vi "EvaluateOperatingStates.vi"(7 "data group":string, 8 "error in (no error)":errorcluster, 9 "map":T1, 10 "config in":T2, 11 "Qbus in":refnum<class "Qbus.lvclass">) -> (0 "error out":errorcluster, 2 "config out":T2, 3 "Qbus out":refnum<class "Qbus.lvclass">)   [LabVIEW 2017, in "OpState.lvlib"]
uses:
  <vilib>/addons/InsightCM/Devices/Shared/Common/OpState/OpState.lvlib
  <vilib>/addons/InsightCM/Devices/Shared/Common/OpState/controls/config.ctl
  <vilib>/addons/Qbus/Qbus.lvclass
  <vilib>/addons/PointValueMap/controls/PointMap.ctl
  <vilib>/addons/InsightCM/Devices/Shared/Common/OpState/controls/ConditionType.ctl
  <vilib>/addons/PointValueMap/subVIs/Point_Write_string.vi
  <vilib>/addons/PointValueMap/PointValueMap.lvlib
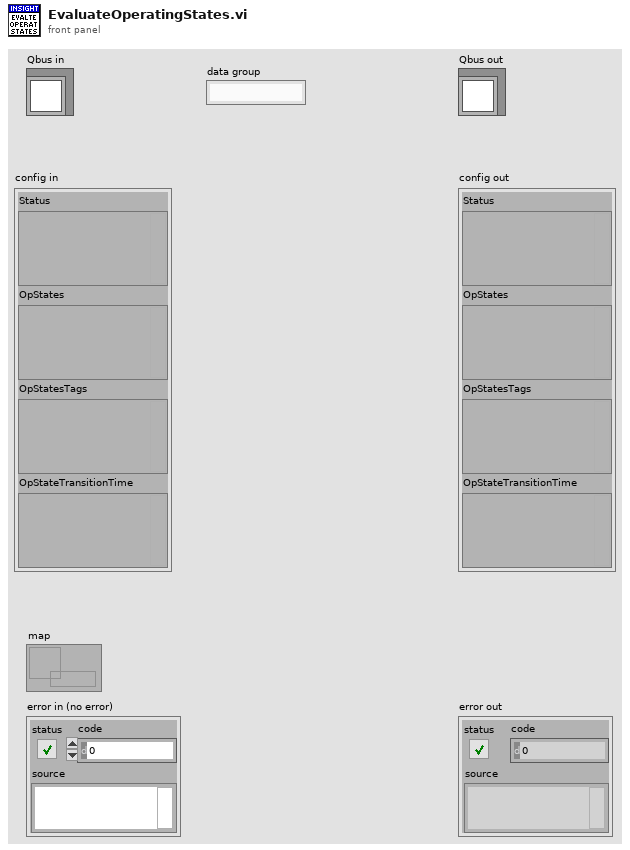
[diagram p1: front panel]
types:
  T1 = typedef "PointValueMap.lvlib/PointMap.ctl" = refnum<data-value>
  T2 = typedef "OpState.lvlib/config.ctl" = cluster{"Status":variant, "OpStates":variant, "OpStatesTags":variant, "OpStateTransitionTime":variant}
  T3 = typedef "OpState.lvlib/ConditionType.ctl" = enum16{"Enter", "Exit"}
  T4 = typedef "Trigger.lvlib/TriggerCondition.ctl" = cluster{"Condition":T5, "LatchValue":string, "LatchTime":timestamp}
  T5 = typedef "Condition.ctl" = cluster{"Source":string, "Type":string, "Operator":string, "CompareTo":string, "DwellSeconds":dbl}
  T6 = typedef "OpState.lvlib/TriggerOperatingState.ctl" = cluster{"Id":string, "Name":string, "Properties":T7[], "EnterExpression":string, "EnterConditions":T4[], "ExitExpression":string, "ExitConditions":T4[]}
  T7 = typedef "KeyValuePair.ctl" = cluster{"Key":string, "Value":string}
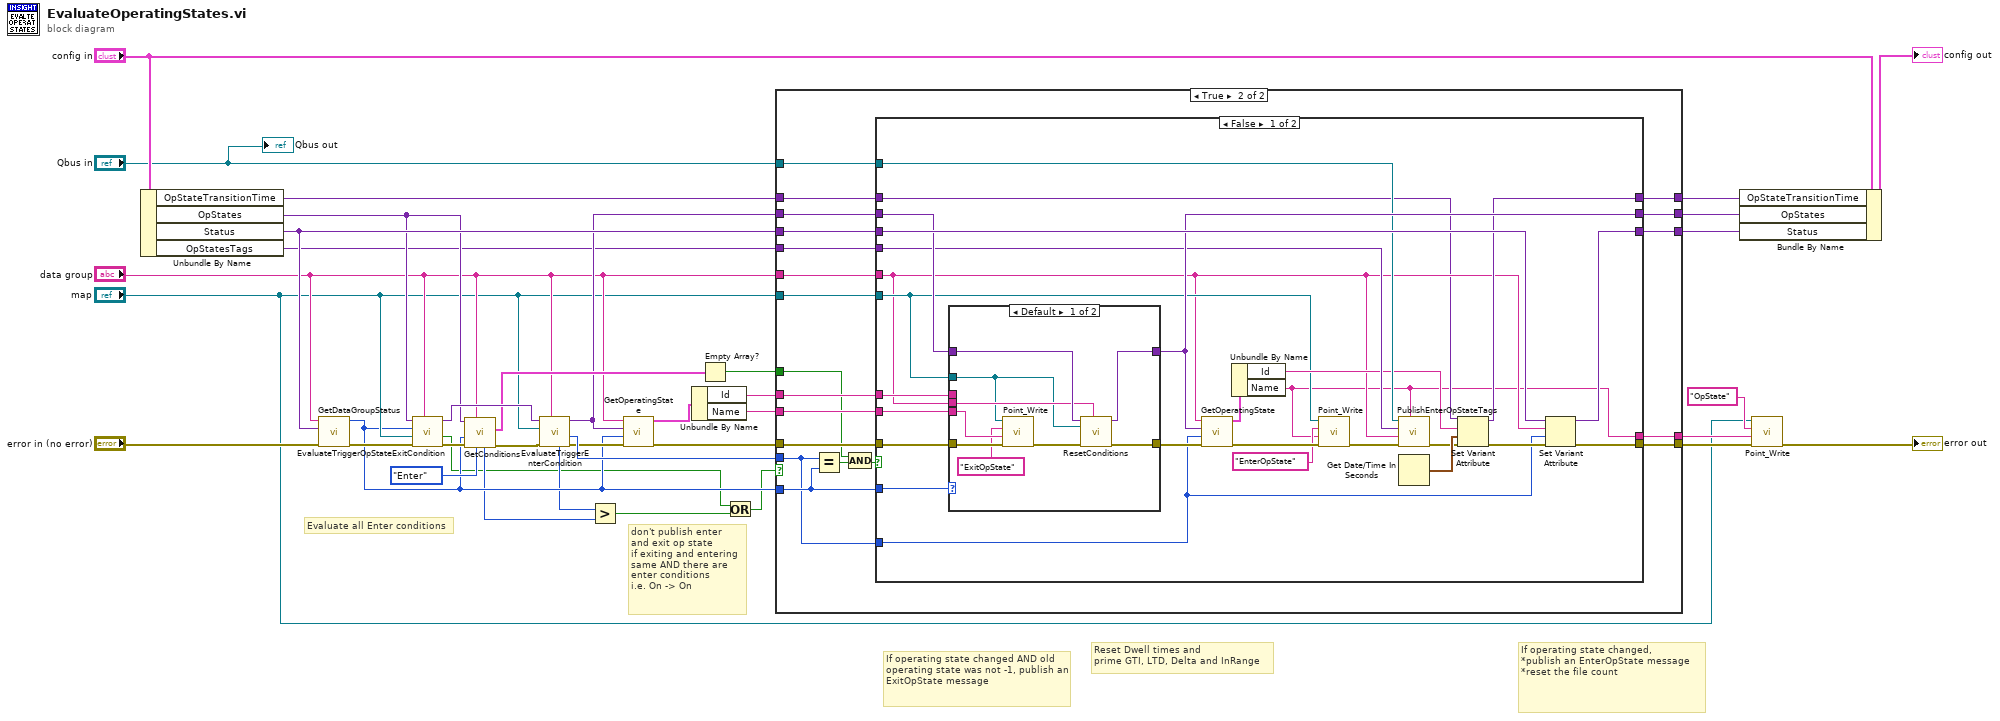
[diagram p0: block diagram]
diagram:
  # "don't publish enter\nand exit op state\nif exiting and entering\nsame AND there are\nenter conditions\ni.e. On -> On"
  # "Reset Dwell times and \nprime GTI, LTD, Delta and InRange"
  # "Evaluate all Enter conditions"
  # "If operating state changed, \n*publish an EnterOpState message\n*reset the file count"
  # "If operating state changed AND old operating state was not -1, publish an ExitOpState message"
  n1 = Unbundle By Name("config in") -> ("OpStateTransitionTime"=w19:variant, "OpStates"=w17:variant, "Status"=w30:variant, "OpStatesTags"=w8:variant)
  n2 = call <vilib>:"GetDataGroupStatus.vi"("error in"="error in (no error)", "status"=w30, "data group"="data group") -> ("error out"=w28:errorcluster, "CurrentOpState"=w7:i32)  [unwired: 7 in]
  n3 = call <vilib>:"EvaluateTriggerOpStateExitCondition.vi"("data group"="data group", "error in"=w28, "map"="map", "current op state"=w7, "operating states in"=w17) -> ("error out"=w13:errorcluster, "exit"=w3:bool, "operating states out"=w33:variant)  [unwired: 4 in]
  n4 = call <vilib>:"GetConditions.vi"("condition type"=ConditionType."Enter", "data group"="data group", "error in (no error)"=w13, "operating state"=w7, "operating states in"=w17) -> ("error out"=w12:errorcluster, "conditions"=w15:T4[], "weight"=w5:i32)  [unwired: 2 in, 2 out]
  n5 = call <vilib>:"EvaluateTriggerEnterCondition.vi"("data group"="data group", "error in"=w12, "map"="map", "operating states in"=w33) -> ("error out"=w23:errorcluster, "new operating state"=w32:i32, "operating states out"=w11:variant, "weight"=w6:i32)  [unwired: 4 in]
  n6 = Greater?(x=w6, y=w5) -> (0:w4:bool)
  n7 = call <vilib>:"GetOperatingState.vi"("error in"=w23, "index"=w7, "operating states"=w11, "data group"="data group") -> ("error out"=w1:errorcluster, "operating state"=w22:T6)  [unwired: 6 in]
  n8 = Unbundle By Name(w22) -> ("Id"=w20:string, "Name"=w21:string)
  n9 = Empty Array?(array=w15) -> (empty?=w14:bool)
  n10 = Or(x=w3, y=w4) -> (x .or. y?=w2:bool)
  n11 = case shown="True" w2 {
    tunnel: w1 -> [w40 w55]
    tunnel: [w40 w62] -> w26
    tunnel: "Qbus in" -> [_ w59]
    tunnel: w11 -> [w41 w54]
    tunnel: "data group" -> [_ w61]
    tunnel: w7 -> [_ w60]
    tunnel: w30 -> [w42 w58]
    tunnel: [w42 w57] -> w34
    tunnel: [w41 w56] -> w35
    tunnel: w32 -> [_ w53]
    tunnel: "map" -> [_ w52]
    tunnel: [w39 w50] -> w24
    tunnel: w21 -> [w39 w51]
    tunnel: w8 -> [_ w49]
    tunnel: w20 -> [_ w48]
    tunnel: w19 -> [w38 w47]
    tunnel: [w38 w46] -> w18
    tunnel: w14 -> [_ w43]
    frame False {
    }
    frame True {
      n12 = Equal?(x=w53, y=w60) -> (x = y?=w44:bool)
      n13 = Compound Arithmetic op=AND(w43, w44) -> (w45:bool)
      n14 = case shown="False" w45 {
        tunnel: w55 -> [w88 w103]
        tunnel: [w82 w103] -> w62
        tunnel: w61 -> [w65 _]
        tunnel: w54 -> [w81 w104]
        tunnel: w60 -> [w87 _]
        tunnel: w59 -> [w74 _]
        tunnel: w53 -> [w66 _]
        tunnel: w58 -> [w84 w102]
        tunnel: [w83 w102] -> w57
        tunnel: [w80 w104] -> w56
        tunnel: w52 -> [w68 _]
        tunnel: w51 -> [w79 w101]
        tunnel: [w63 w101] -> w50
        tunnel: w49 -> [w75 _]
        tunnel: w48 -> [w76 _]
        tunnel: w47 -> [w64 w100]
        tunnel: [w69 w100] -> w46
        frame False {
          n15 = case shown="Default" w87 {
            tunnel: w88 -> [w93 w99]
            tunnel: w65 -> [w94 _]
            tunnel: w81 -> [w96 w98]
            tunnel: [w97 w99] -> w86
            tunnel: [w95 w98] -> w80
            tunnel: w68 -> [w90 _]
            tunnel: w79 -> [w92 _]
            tunnel: w76 -> [_ _]
            frame Default {
              n16 = call-poly <vilib>:"Point_Write.vi"("Error In"=w93, "Value"=w92, "Tag"="ExitOpState", "Map"=w90) -> ("Error Out"=w89:errorcluster)  [unwired: 6 in, 1 out]
              n17 = call <vilib>:"ResetConditions.vi"("data group"=w94, "error in (no error)"=w89, "map"=w90, "operating states in"=w96) -> ("error out"=w97:errorcluster, "operating states out"=w95:variant)  [unwired: 6 in]
            }
            frame -1 {
            }
          }
          n18 = call <vilib>:"GetOperatingState.vi"("error in"=w86, "index"=w66, "operating states"=w80, "data group"=w65) -> ("error out"=w78:errorcluster, "operating state"=w85:T6)  [unwired: 6 in]
          n19 = Unbundle By Name(w85) -> ("Id"=w73:string, "Name"=w63:string)
          n20 = call-poly <vilib>:"Point_Write.vi"("Error In"=w78, "Value"=w63, "Tag"="EnterOpState", "Map"=w68) -> ("Error Out"=w67:errorcluster)  [unwired: 6 in, 1 out]
          n21 = call <vilib>:"PublishEnterOpStateTags.vi"("op state"=w63, "error in (no error)"=w67, "data group name"=w65, "operating states tags"=w75, "Qbus in"=w74) -> ("error out"=w71:errorcluster)  [unwired: 6 in]
          n22 = Get Date/Time In Seconds() -> (seconds since 1Jan1904=w72:timestamp)
          n23 = Set Variant Attribute(Variant=w64, name=w73, value=w72, error in=w71) -> (Variant out=w69:variant, error out=w70:errorcluster)  [unwired: 1 out]
          n24 = Set Variant Attribute(Variant=w84, name=w65, value=w66, error in=w70) -> (Variant out=w83:variant, error out=w82:errorcluster)  [unwired: 1 out]
        }
        frame True {
        }
      }
    }
  }
  n25 = Bundle By Name(cluster="config in", "OpStateTransitionTime"=w18, "OpStates"=w35, "Status"=w34) -> (→"config out":T2)
  n26 = call-poly <vilib>:"Point_Write.vi"("Error In"=w26, "Value"=w24, "Tag"="OpState", "Map"="map") -> ("Error Out"=→"error out":errorcluster)  [unwired: 6 in, 1 out]
  "Qbus out" <- "Qbus in"
